vi "Abbreviator.vi"(9 "replaceArray":cluster{"find":string, "replace":string}[](array[cluster]), 10 "Max String Length (0)":i32, 11 "longStringIn":string) -> (0 "stillTooLong":bool, 2 "finalLength":i32, 3 "shortStringOut":string, 5 "audit":string[](array[string]))   [LabVIEW 2020]
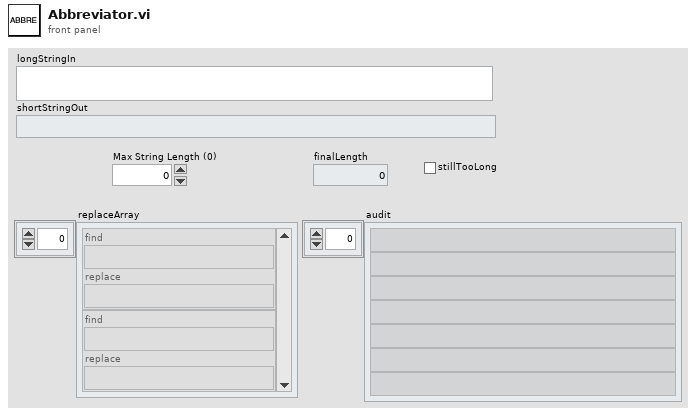
[diagram p1: front panel]
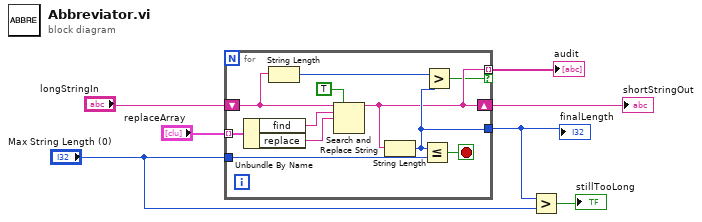
[diagram p0: block diagram]
diagram:
  n1 = for {
    shift-right: [w9] -> w7
    shift-left: "longStringIn" -> [w12]
    tunnel: "replaceArray" -> [w17] mode=indexing
    tunnel: "Max String Length (0)" -> [w14]
    tunnel: [w10] -> w4
    tunnel: [w9] -> w1 mode=indexing if=w8
    stop <- w13 stop-if-true
    n2 = Unbundle By Name(w17) -> ("find"=w16:string, "replace"=w15:string)
    n3 = String Length(string=w12) -> (length=w11:i32)
    n4 = Search and Replace String(replace all?=TRUE ("replace all? (F)"), input string=w12, search string=w16, replace string=w15) -> (result string=w9:string)  [unwired: 4 in, 3 out]
    n5 = String Length(string=w9) -> (length=w10:i32)
    n6 = Less Or Equal?(x=w10, y=w14) -> (x <= y?=w13:bool)
    n7 = Greater?(x=w11, y=w10) -> (0:w8:bool)
  }
  "shortStringOut" <- w7
  "finalLength" <- w4
  "audit" <- w1
  n8 = Greater?(x=w4, y="Max String Length (0)") -> (0:→"stillTooLong":bool)
